vi "niccc-labview.vi"() -> ()   [LabVIEW 2020]
uses:
  Controls/Frame Info.ctl
  Controls/Vertex.ctl
  Controls/State.ctl
panel:
  in  "FPS":u32=20
  in  "Wireframe":bool
  in  "Slow Draw":bool
  out "Frame":i32
  out "Canvas":picture
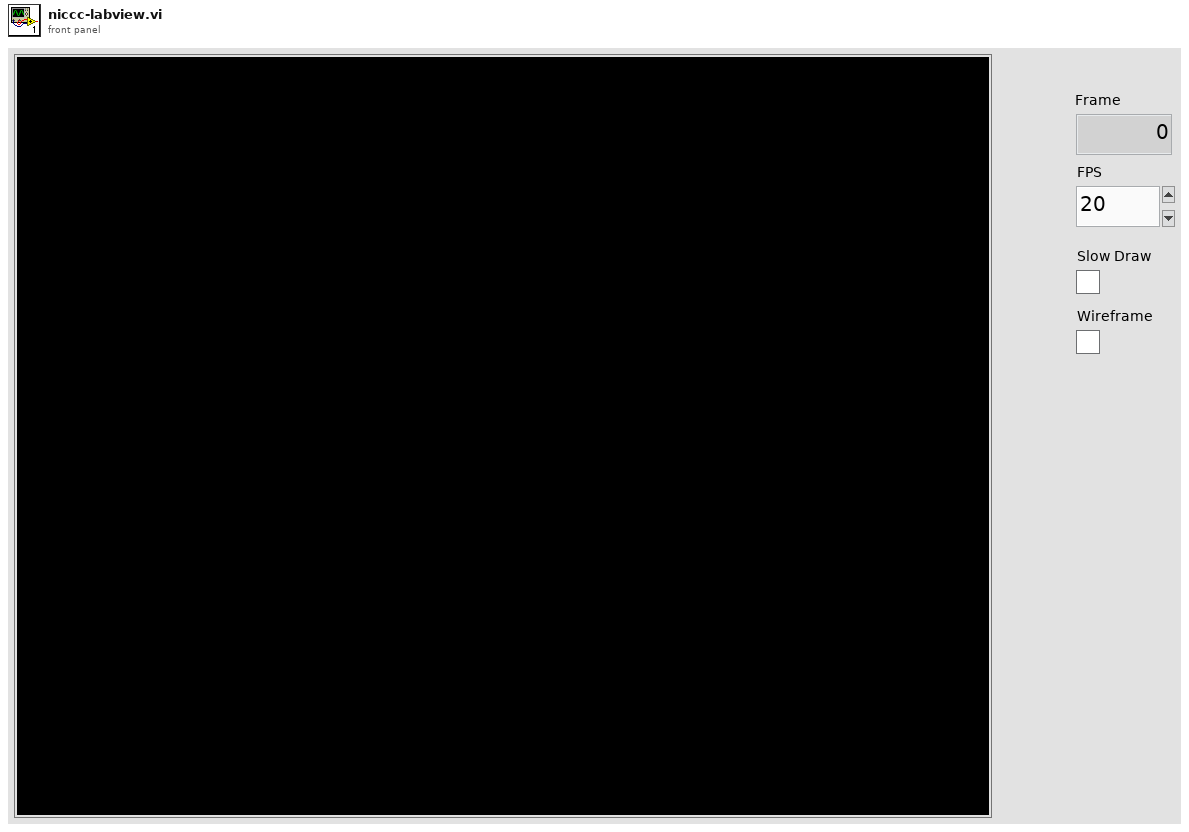
[diagram p1: front panel]
types:
  T1 = typedef "Frame Info.ctl" = cluster{"Clear Screen":bool, "Palette Data":bool, "Indexed":bool, "Canvas":picture, "Palette":u32[], "Indexed Verts":T2[], "Frame":i32}
  T2 = typedef "Vertex.ctl" = cluster{"x":u8, "y":u8}
  T3 = typedef "State.ctl" = enum16{"Init", "Read Flags", "Clear Screen", "Update Palette", "Read Indexed", "Draw Polygons", "Skip 64kB", "Finish"}
  T4 = cluster{"left":i16, "top":i16, "right":i16, "bottom":i16}
  T5 = cluster{"Width":u16, "Style":enum32{"Solid", "Dash", "Dot", "DashDot", "DashDotDot"}}
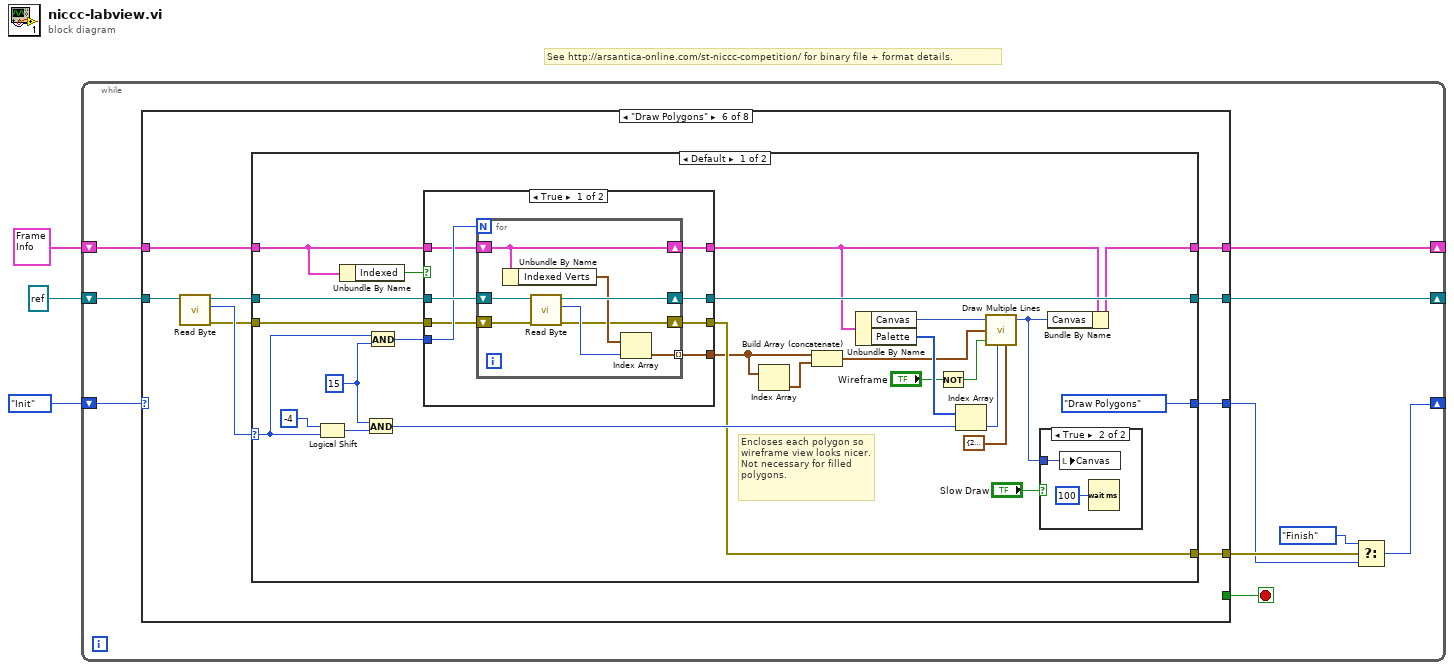
[diagram p0: block diagram]
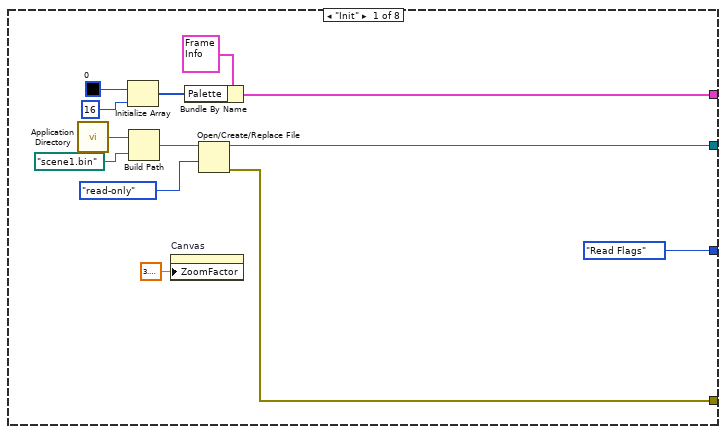
[diagram p2: hidden frame]
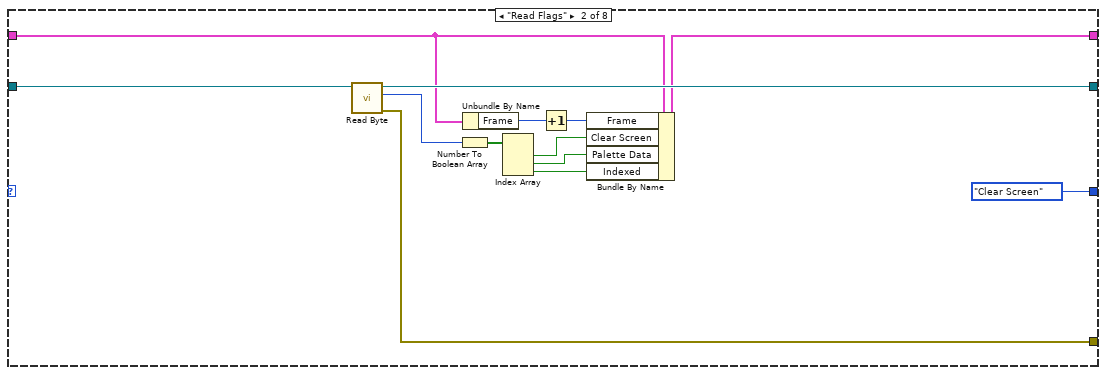
[diagram p3: hidden frame]
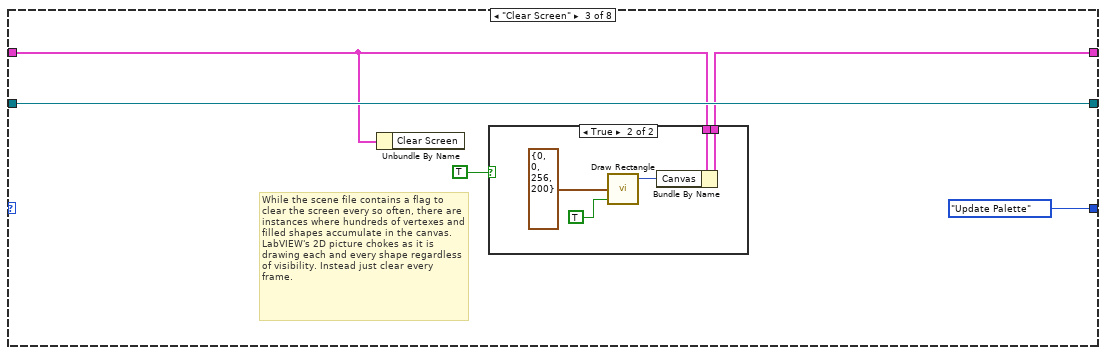
[diagram p4: hidden frame]
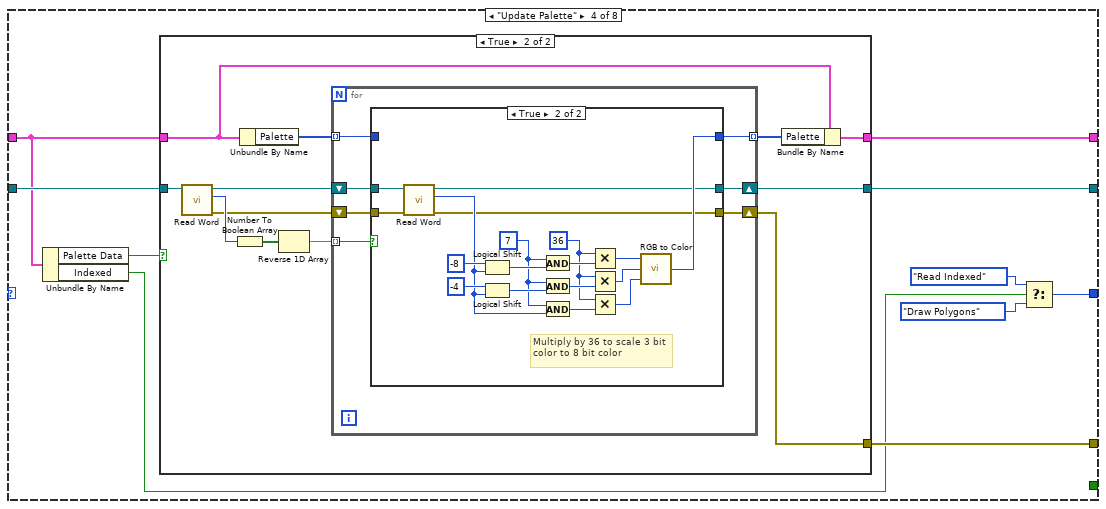
[diagram p6: hidden frame]
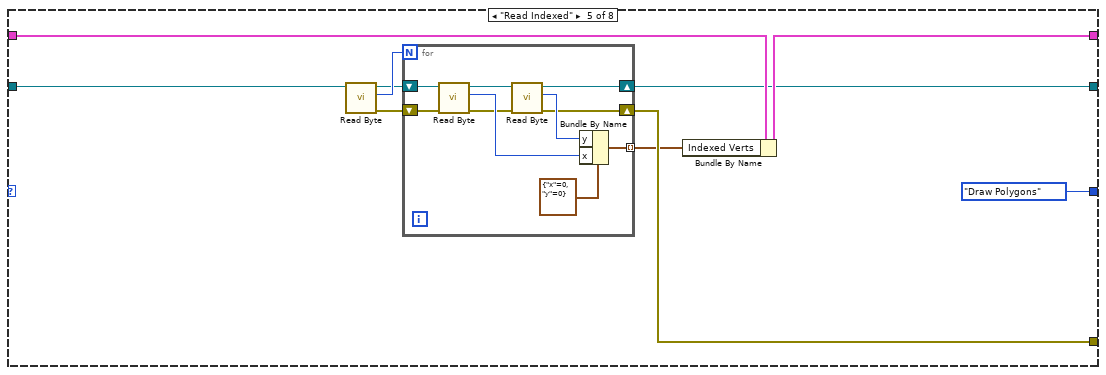
[diagram p9: hidden frame]
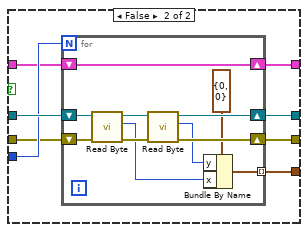
[diagram p11: hidden frame]
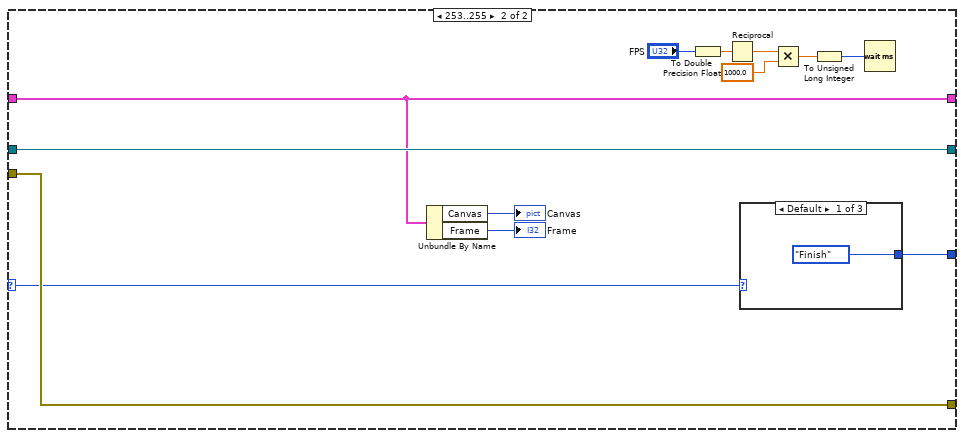
[diagram p12: hidden frame]
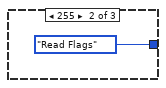
[diagram p13: hidden frame]
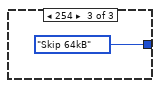
[diagram p14: hidden frame]
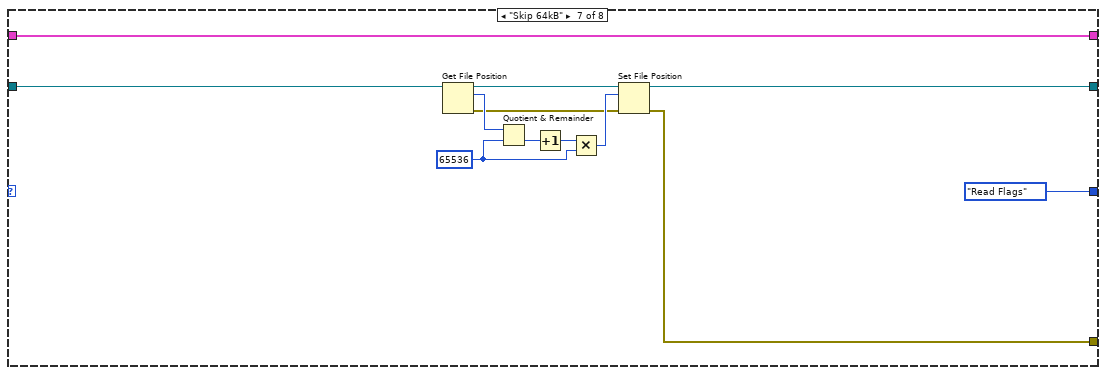
[diagram p15: hidden frame]
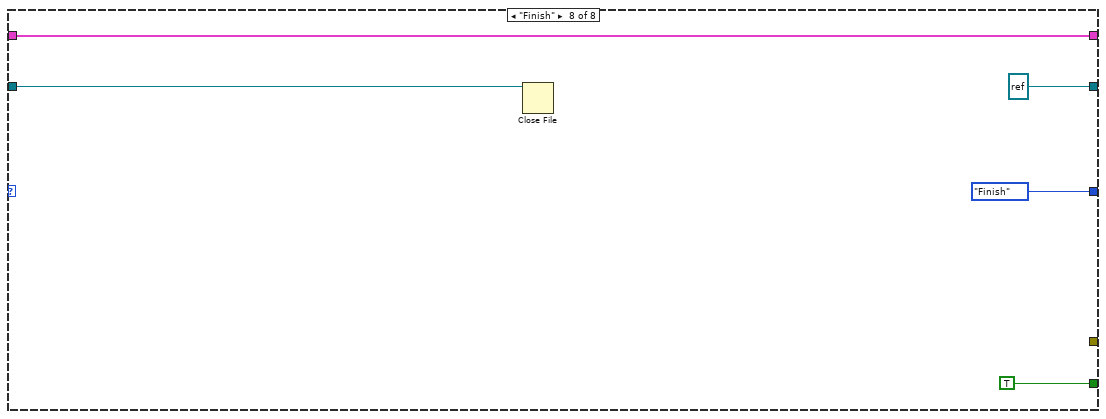
[diagram p16: hidden frame]
diagram:
  # "See http://arsantica-online.com/st-niccc-competition/ for binary file + format details."
  n1 = while {
    shift-right: [w5] -> _
    shift-left: State."Init" -> [w13]
    shift-right: [w12] -> _
    shift-left: refnum<file> refnum ("refnum out") -> [w11]
    shift-right: [w9] -> _
    shift-left: T1 {"Clear Screen"=FALSE, "Palette Data"=FALSE, "Indexed"=FALSE, "Canvas"=bytes[0], "Palette"=[], "Indexed Verts"=[], "Frame"=0} -> [w10]
    stop <- w4 stop-if-true
    n2 = case shown="\"Draw Polygons\"" w13 {
      tunnel: [w22 w38 w44 w59 w107 w125 w217 refnum<file> refnum ("refnum out")] -> w12
      tunnel: w11 -> [_ w39 w44 w60 w112 w131 w218 w227]
      tunnel: w10 -> [_ w29 w42 w53 w108 w127 w222 w226]
      tunnel: [w20 w33 w43 w58 w109 w126 w222 w226] -> w9
      tunnel: [State."Read Flags" State."Clear Screen" State."Update Palette" w54 State."Draw Polygons" w129 State."Read Flags" State."Finish"] -> w6
      tunnel: [w16 w32 _ w57 w105 w123 w211 _] -> w7
      tunnel: [_ _ _ _ _ _ _ TRUE] -> w4
      frame "Init" {
        n3 = call <vilib>:"Application Directory.vi"() -> ("Application Directory"=w26:path)
        n4 = Initialize Array(u32 0, 16) -> (w18:u32[])
        n5 = Build Path(base path=w26, name or relative path=path "scene1.bin") -> (appended path=w24:path)
        n6 = property on="Canvas" class="Pict"("ZoomFactor"=sgl 3.8 ("Zoom Factor")) -> ()  [unwired: 2 in, 2 out]
        n7 = Bundle By Name(cluster=T1 {"Clear Screen"=FALSE, "Palette Data"=FALSE, "Indexed"=FALSE, "Canvas"=bytes[0], "Palette"=[], "Indexed Verts"=[], "Frame"=0}, "Palette"=w18) -> (w20:T1)
        n8 = Open/Create/Replace File(file path (use dialog)=w24, access (0:read/write)=enum16{"read/write", "read-only", "write-only"}."read-only") -> (refnum out=w22:refnum<file>, error out=w16:errorcluster)  [unwired: 4 in, 1 out]
      }
      frame "Read Flags" {
        n9 = call "Read Byte.vi"("File Ref In"=w39) -> ("error out"=w32:errorcluster, "Word"=w37:u8, "File Ref Out"=w38:refnum<file>)  [unwired: 8 in]
        n10 = Number To Boolean Array(number=w37) -> (Boolean array=w36:bool[])
        n11 = Unbundle By Name(w29) -> ("Frame"=w28:i32)
        n12 = Index Array(array=w36) -> (element #1=w31:bool, element #2=w35:bool, element #3=w34:bool)  [unwired: 3 in]
        n13 = Increment(x=w28) -> (x+1=w27:i32)
        n14 = Bundle By Name(cluster=w29, "Frame"=w27, "Clear Screen"=w31, "Palette Data"=w35, "Indexed"=w34) -> (w33:T1)
      }
      frame "Clear Screen" {
        # "While the scene file contains a flag to clear the screen every so often, there are instances where hundreds of vertexes and filled shapes accumulate in the canvas. LabVIEW's 2D picture chokes as it is drawing each and every shape regardless of visibility. Instead just clear every frame."
        n15 = Unbundle By Name(w42) -> ()  [unwired: 1 out]
        n16 = case shown="True" TRUE {
          tunnel: w42 -> [w45 w50]
          tunnel: [w45 w49] -> w43
          frame False {
          }
          frame True {
            n17 = call <vilib>:"Draw Rectangle.vi"("rect"=T4 {"left"=0, "top"=0, "right"=256, "bottom"=200}, "fill?(F)"=TRUE) -> ("new picture"=w48:picture)  [unwired: 7 in]
            n18 = Bundle By Name(cluster=w50, "Canvas"=w48) -> (w49:T1)
          }
        }
      }
      frame "Update Palette" {
        n19 = Unbundle By Name(w53) -> ("Palette Data"=w52:bool, "Indexed"=w51:bool)
        n20 = case shown="True" w52 {
          tunnel: w60 -> [w61 w74]
          tunnel: [w61 w70] -> w59
          tunnel: w53 -> [w62 w67]
          tunnel: [w62 w66] -> w58
          tunnel: [_ w63] -> w57
          frame False {
          }
          frame True {
            n21 = call "Read Word.vi"("File Ref In"=w74) -> ("error out"=w64:errorcluster, "Word"=w73:u16, "File Ref Out"=w71:refnum<file>)  [unwired: 8 in]
            n22 = Number To Boolean Array(number=w73) -> (Boolean array=w72:bool[])
            n23 = Unbundle By Name(w67) -> ("Palette"=w69:u32[])
            n24 = Reverse 1D Array(array=w72) -> (reversed array=w68:bool[])
            n25 = for {
              tunnel: w68 -> [w79] mode=indexing
              shift-right: [w77] -> w70
              shift-left: w71 -> [w81]
              tunnel: w69 -> [w80] mode=indexing
              tunnel: [w78] -> w65 mode=indexing
              shift-right: [w75] -> w63
              shift-left: w64 -> [w76]
              n26 = case shown="True" w79 {
                tunnel: w81 -> [w83 w102]
                tunnel: w80 -> [w84 _]
                tunnel: [w84 w101] -> w78
                tunnel: [w83 w87] -> w77
                tunnel: w76 -> [w82 w86]
                tunnel: [w82 w85] -> w75
                frame False {
                }
                frame True {
                  w91 = u16 36 ("x")
                  w96 = u16 7 ("y")
                  # "Multiply by 36 to scale 3 bit color to 8 bit color"
                  n27 = call "Read Word.vi"("error in"=w86, "File Ref In"=w102) -> ("error out"=w85:errorcluster, "Word"=w95:u16, "File Ref Out"=w87:refnum<file>)  [unwired: 7 in]
                  n28 = Logical Shift(y=-8 ("x"), x=w95) -> (x << y=w98:u16)
                  n29 = Logical Shift(y=-4 ("x"), x=w95) -> (x << y=w97:u16)
                  n30 = And(x=w96, y=w98) -> (x .and. y?=w94:u16)
                  n31 = And(x=w96, y=w97) -> (x .and. y?=w92:u16)
                  n32 = And(x=w96, y=w95) -> (x .and. y?=w90:u16)
                  n33 = Multiply(x=w91, y=w94) -> (x*y=w93:u16)
                  n34 = Multiply(x=w91, y=w92) -> (x*y=w89:u16)
                  n35 = Multiply(x=w91, y=w90) -> (x*y=w88:u16)
                  n36 = call <vilib>:"RGB to Color.vi"("B"=w88, "G"=w89, "R"=w93) -> ("Color"=w101:u32)
                }
              }
            }
            n37 = Bundle By Name(cluster=w67, "Palette"=w65) -> (w66:T1)
          }
        }
        n38 = Select(t=State."Read Indexed", s=w51, f=State."Draw Polygons") -> (s? t:f=w54:T3)
      }
      frame "Read Indexed" {
        n39 = call "Read Byte.vi"("File Ref In"=w112) -> ("error out"=w106:errorcluster, "Word"=w111:u8, "File Ref Out"=w110:refnum<file>)  [unwired: 8 in]
        n40 = for {
          N: w111 -> [_]
          shift-right: [w120] -> w107
          shift-left: w110 -> [w122]
          tunnel: [w119] -> w103 mode=indexing
          shift-right: [w113] -> w105
          shift-left: w106 -> [w115]
          n41 = call "Read Byte.vi"("error in"=w115, "File Ref In"=w122) -> ("error out"=w114:errorcluster, "Word"=w117:u8, "File Ref Out"=w121:refnum<file>)  [unwired: 7 in]
          n42 = call "Read Byte.vi"("error in"=w114, "File Ref In"=w121) -> ("error out"=w113:errorcluster, "Word"=w116:u8, "File Ref Out"=w120:refnum<file>)  [unwired: 7 in]
          n43 = Bundle By Name(cluster=T2 {"x"=0, "y"=0}, "y"=w116, "x"=w117) -> (w119:T2)
        }
        n44 = Bundle By Name(cluster=w108, "Indexed Verts"=w103) -> (w109:T1)
      }
      frame "Draw Polygons" {
        n45 = call "Read Byte.vi"("File Ref In"=w131) -> ("error out"=w124:errorcluster, "Word"=w130:u8, "File Ref Out"=w128:refnum<file>)  [unwired: 8 in]
        n46 = case shown="Default" w130 {
          selector: w130 -> [w154 w203]
          tunnel: [State."Draw Polygons" w207] -> w129
          tunnel: w128 -> [w149 w206]
          tunnel: w127 -> [w142 w205]
          tunnel: [w147 w205] -> w126
          tunnel: [w150 w206] -> w125
          tunnel: w124 -> [w144 w204]
          tunnel: [w143 w204] -> w123
          frame Default {
            w153 = u8 15 ("y")
            # "Encloses each polygon so wireframe view looks nicer. Not necessary for filled polygons."
            n47 = Logical Shift(y=i16 -4, x=w154) -> (x << y=w156:u8)
            n48 = Unbundle By Name(w142) -> ("Indexed"=w141:bool)
            n49 = And(x=w153, y=w156) -> (x .and. y?=w152:u8)
            n50 = And(x=w154, y=w153) -> (x .and. y?=w148:u8)
            n51 = case shown="True" w141 {
              tunnel: [w167 w183] -> w150
              tunnel: w149 -> [w166 w182]
              tunnel: w148 -> [w165 w181]
              tunnel: w142 -> [w164 w180]
              tunnel: [w163 w179] -> w134
              tunnel: [w162 w178] -> w146
              tunnel: w144 -> [w161 w177]
              tunnel: [w160 w176] -> w143
              frame True {
                n52 = for {
                  N: w165 -> [_]
                  shift-right: [w174] -> w167
                  shift-left: w166 -> [w175]
                  shift-right: [w171] -> w162
                  shift-left: w164 -> [w171]
                  tunnel: [w170] -> w163 mode=indexing
                  shift-right: [w168] -> w160
                  shift-left: w161 -> [w169]
                  n53 = Unbundle By Name(w171) -> ("Indexed Verts"=w173:T2[])
                  n54 = call "Read Byte.vi"("error in"=w169, "File Ref In"=w175) -> ("error out"=w168:errorcluster, "Word"=w172:u8, "File Ref Out"=w174:refnum<file>)  [unwired: 7 in]
                  n55 = Index Array(array=w173, index=w172) -> (element=w170:T2)
                }
              }
              frame False {
                n56 = for {
                  N: w181 -> [_]
                  shift-right: [w190] -> w183
                  shift-left: w182 -> [w194]
                  shift-right: [w193] -> w178
                  shift-left: w180 -> [w193]
                  tunnel: [w184] -> w179 mode=indexing
                  shift-right: [w189] -> w176
                  shift-left: w177 -> [w192]
                  n57 = call "Read Byte.vi"("error in"=w192, "File Ref In"=w194) -> ("error out"=w188:errorcluster, "Word"=w185:u8, "File Ref Out"=w191:refnum<file>)  [unwired: 7 in]
                  n58 = call "Read Byte.vi"("error in"=w188, "File Ref In"=w191) -> ("error out"=w189:errorcluster, "Word"=w186:u8, "File Ref Out"=w190:refnum<file>)  [unwired: 7 in]
                  n59 = Bundle By Name(cluster=T2 {"x"=0, "y"=0} ("Vertex"), "y"=w186, "x"=w185) -> (w184:T2)
                }
              }
            }
            n60 = Index Array(array=w134) -> (element=w133:T2)  [unwired: 1 in]
            n61 = Build Array (concatenate)(w134, w133) -> (w132:T2[])
            n62 = Unbundle By Name(w146) -> ("Canvas"=w135:picture, "Palette"=w145:u32[])
            n63 = Not(x="Wireframe") -> (.not. x?=w137:bool)
            n64 = Index Array(array=w145, index=w152) -> (element=w151:u32)
            n65 = call <vilib>:"Draw Multiple Lines.vi"("picture"=w135, "line endpoints"=w132, "fill?(F)"=w137, "color(black)"=w151, "pen"=T5 {"Width"=2, "Style"=enum."Solid"}) -> ("new picture"=w140:picture)  [unwired: 4 in]
            n66 = case shown="True" "Slow Draw" {
              tunnel: w140 -> [_ w159]
              frame False {
              }
              frame True {
                n67 = local write "Canvas"(w159) -> ()
                n68 = Wait (ms)(milliseconds to wait=u32 100) -> ()  [unwired: 1 out]
              }
            }
            n69 = Bundle By Name(cluster=w146, "Canvas"=w140) -> (w147:T1)
          }
          frame 253..255 {
            n70 = Unbundle By Name(w205) -> ("Canvas"=→"Canvas":picture, "Frame"=→"Frame":i32)
            n71 = To Double Precision Float(number="FPS") -> (double precision float=w201:dbl)
            n72 = Reciprocal(x=w201) -> (1/x=w197:dbl)
            n73 = case shown="Default" w203 {
              tunnel: [State."Finish" State."Read Flags" State."Skip 64kB"] -> w207
              frame Default {
              }
              frame 255 {
              }
              frame 254 {
              }
            }
            n74 = Multiply(x=w197, y=1000.0) -> (x*y=w199:dbl)
            n75 = To Unsigned Long Integer(number=w199) -> (unsigned 32bit integer=w196:u32)
            n76 = Wait (ms)(milliseconds to wait=w196) -> ()  [unwired: 1 out]
          }
        }
      }
      frame "Skip 64kB" {
        w214 = i64 65536 ("y")
        n77 = Get File Position(7:w218) -> (0:w212:errorcluster, 2:w220:i64, 3:w219:refnum<file>)  [unwired: 1 in]
        n78 = Quotient & Remainder(x=w220, y=w214) -> (floor(x/y)=w216:i64)  [unwired: 1 out]
        n79 = Increment(x=w216) -> (x+1=w215:i64)
        n80 = Multiply(x=w215, y=w214) -> (x*y=w213:i64)
        n81 = Set File Position(offset (in bytes) (0)=w213, refnum=w219, error in=w212) -> (refnum out=w217:refnum<file>, error out=w211:errorcluster)  [unwired: 1 in]
      }
      frame "Finish" {
        n82 = Close File(refnum=w227) -> ()  [unwired: 1 in, 2 out]
      }
    }
    n83 = Select(t=State."Finish", s=w7, f=w6) -> (s? t:f=w5:T3)
  }
